vi "EnFlo_TubingCorrection_Sub.vi"(4 "Index":i32, 5 "Analysis Info cluster In":T1={"Colour"=0, "Inst type"=enum."Pitot-static tube", "Inst name"="Manometer voltage", "Symbol"="U", "Code name"="", "Extra Info"="U", "Inst Array"=enum."PWA", "U"=0.0, "u^2"=0.0, "u^3"=0.0, "u^4"=0.0, "Skew_u"=0.0, "Kurt_u"=0.0, "Sd Error in Mean"=0.0, "% u'/U"=0.0, "X"=0.0, "Y"=0.0, "Z"=0.0, "Timescale integral Estimate"=0.0, "Sd Error in Variance"=0.0, "Calib File"=path "", "Calib Constants"=[], "Output Position"=FALSE, "Stats"=enum."None", "Av Sampling Rate"=0.0, "Av No of Samples"=0.0, "Total Meas Time (s)"=0.0, "OrigChName"="", "Max value"=0.0, "Min value"=0.0, "Req Sample Rate Hz"=0.0, "Sync Delay Time (s)"=0.0, "Ch No"=0, "Device"="", "Use Latest Calib"=FALSE, "Port"="", "Metadata Ch Names"=[], "Metadata Ch Values"=[], "Label"="", "chState"=enum."No Selection", "Point Drift"=0.0, "inputConfig"=""} {"Kurt_u" format="%_3g"; "u^4" format="%_3g"; "u^3" format="%_3g"; "Sd Error in Variance" format="%_3g"; "u^2" format="%_3g"; "Sd Error in Mean" format="%_3g"; "U" format="%_3g"; "Sync Delay Time (s)" format="%.4f"; "Total Meas Time (s)" format="%_5g"; "Skew_u" format="%_3g"; "% u'/U" format="%_3g"}, 6 "Time Trace In":T5, 7 "Phase":dbl[](array[numeric]), 8 "Gain":dbl[](array[numeric]), 9 "Freq Hz":dbl[](array[numeric])) -> (0 "Time Trace out":T5, 3 "Analysis Info cluster Out":T1={"Colour"=0, "Inst type"=enum."Pitot-static tube", "Inst name"="Manometer voltage", "Symbol"="U", "Code name"="", "Extra Info"="U", "Inst Array"=enum."PWA", "U"=0.0, "u^2"=0.0, "u^3"=0.0, "u^4"=0.0, "Skew_u"=0.0, "Kurt_u"=0.0, "Sd Error in Mean"=0.0, "% u'/U"=0.0, "X"=0.0, "Y"=0.0, "Z"=0.0, "Timescale integral Estimate"=0.0, "Sd Error in Variance"=0.0, "Calib File"=path "", "Calib Constants"=[], "Output Position"=FALSE, "Stats"=enum."None", "Av Sampling Rate"=0.0, "Av No of Samples"=0.0, "Total Meas Time (s)"=0.0, "OrigChName"="", "Max value"=0.0, "Min value"=0.0, "Req Sample Rate Hz"=0.0, "Sync Delay Time (s)"=0.0, "Ch No"=0, "Device"="", "Use Latest Calib"=FALSE, "Port"="", "Metadata Ch Names"=[], "Metadata Ch Values"=[], "Label"="", "chState"=enum."No Selection", "Point Drift"=0.0, "inputConfig"=""} {"Kurt_u" format="%_3g"; "u^4" format="%_3g"; "u^3" format="%_3g"; "Sd Error in Variance" format="%_3g"; "u^2" format="%_3g"; "Sd Error in Mean" format="%_3g"; "U" format="%_3g"; "Sync Delay Time (s)" format="%.4f"; "Total Meas Time (s)" format="%_5g"; "Skew_u" format="%_3g"; "% u'/U" format="%_3g"})   [LabVIEW 2022 SP3]
uses:
  <vilib>/Analysis/NI_AALPro.lvlib
  <vilib>/Analysis/2dsp.llb/Real FFT.vi
  <vilib>/Analysis/2dsp.llb/Inverse Real FFT.vi
  <vilib>/Analysis/NI_AALBase.lvlib
  <vilib>/Analysis/baseanly.llb/Mean (DBL).vi
  Globals/Meas_global.vi
  Controls/Time_Trace_Cluster.ctl
  Controls/Inst_type.ctl
  Controls/Instrument_Array.ctl
  Controls/Analysis_info_cluster.ctl
  Controls/channelState.ctl
panel:
  out "N Smoothing":i32
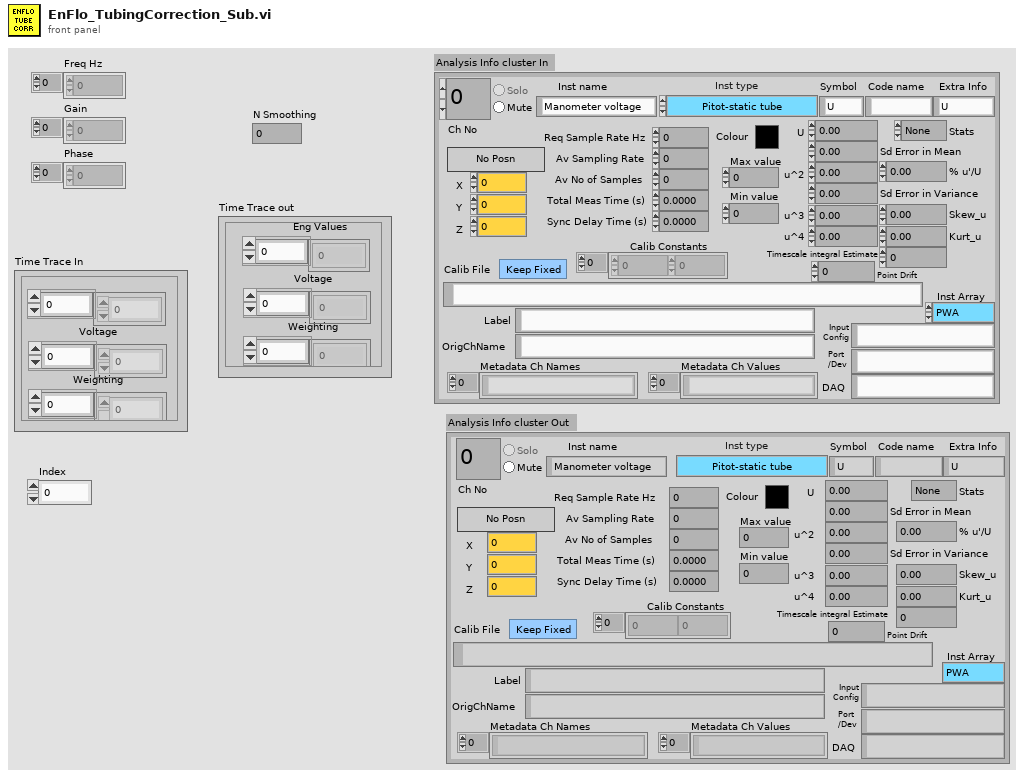
[diagram p1: front panel]
types:
  T1 = typedef "Analysis_info_cluster.ctl" = cluster{"Colour":u32, "Inst type":T2, "Inst name":string, "Symbol":string, "Code name":string, "Extra Info":string, "Inst Array":T3, "U":dbl, "u^2":dbl, "u^3":dbl, "u^4":dbl, "Skew_u":dbl, "Kurt_u":dbl, "Sd Error in Mean":dbl, "% u'/U":dbl, "X":dbl, "Y":dbl, "Z":dbl, "Timescale integral Estimate":dbl, "Sd Error in Variance":dbl, "Calib File":path, "Calib Constants":dbl[], "Output Position":bool, "Stats":enum16{"None", "Basic", "Full"}, "Av Sampling Rate":dbl, "Av No of Samples":dbl, "Total Meas Time (s)":dbl, "OrigChName":string, "Max value":dbl, "Min value":dbl, "Req Sample Rate Hz":dbl, "Sync Delay Time (s)":dbl, "Ch No":i16, "Device":string, "Use Latest Calib":bool, "Port":string, "Metadata Ch Names":string[], "Metadata Ch Values":string[], "Label":string, "chState":T4, "Point Drift":dbl, "inputConfig":string}
  T2 = typedef "Inst_type.ctl" = enum16{"Raw voltage", "Raw with zero offsetting", "Propeller anemometer", "Pressure Transducer", "Pitot-static tube", "Hot wire", "Cross wire 1", "Cross wire 2", "Generic Linear", "Generic Polynomial", "Generic BackPoly", "Fast FID", "Thermocouple", "Cold wire", "Pulsed Wire", "LDA Vel", "LDA Tran time", "LDA Arr time", "Microphone"}
  T3 = typedef "Instrument_Array.ctl" = enum16{"PWA", "LDA", "Analogue"}
  T4 = typedef "channelState.ctl" = enum32{"No Selection", "Solo", "Mute"}
  T5 = typedef "Time_Trace_Cluster.ctl" = cluster{"Weighting":dbl[], "Voltage":dbl[], "Eng Values":dbl[]}
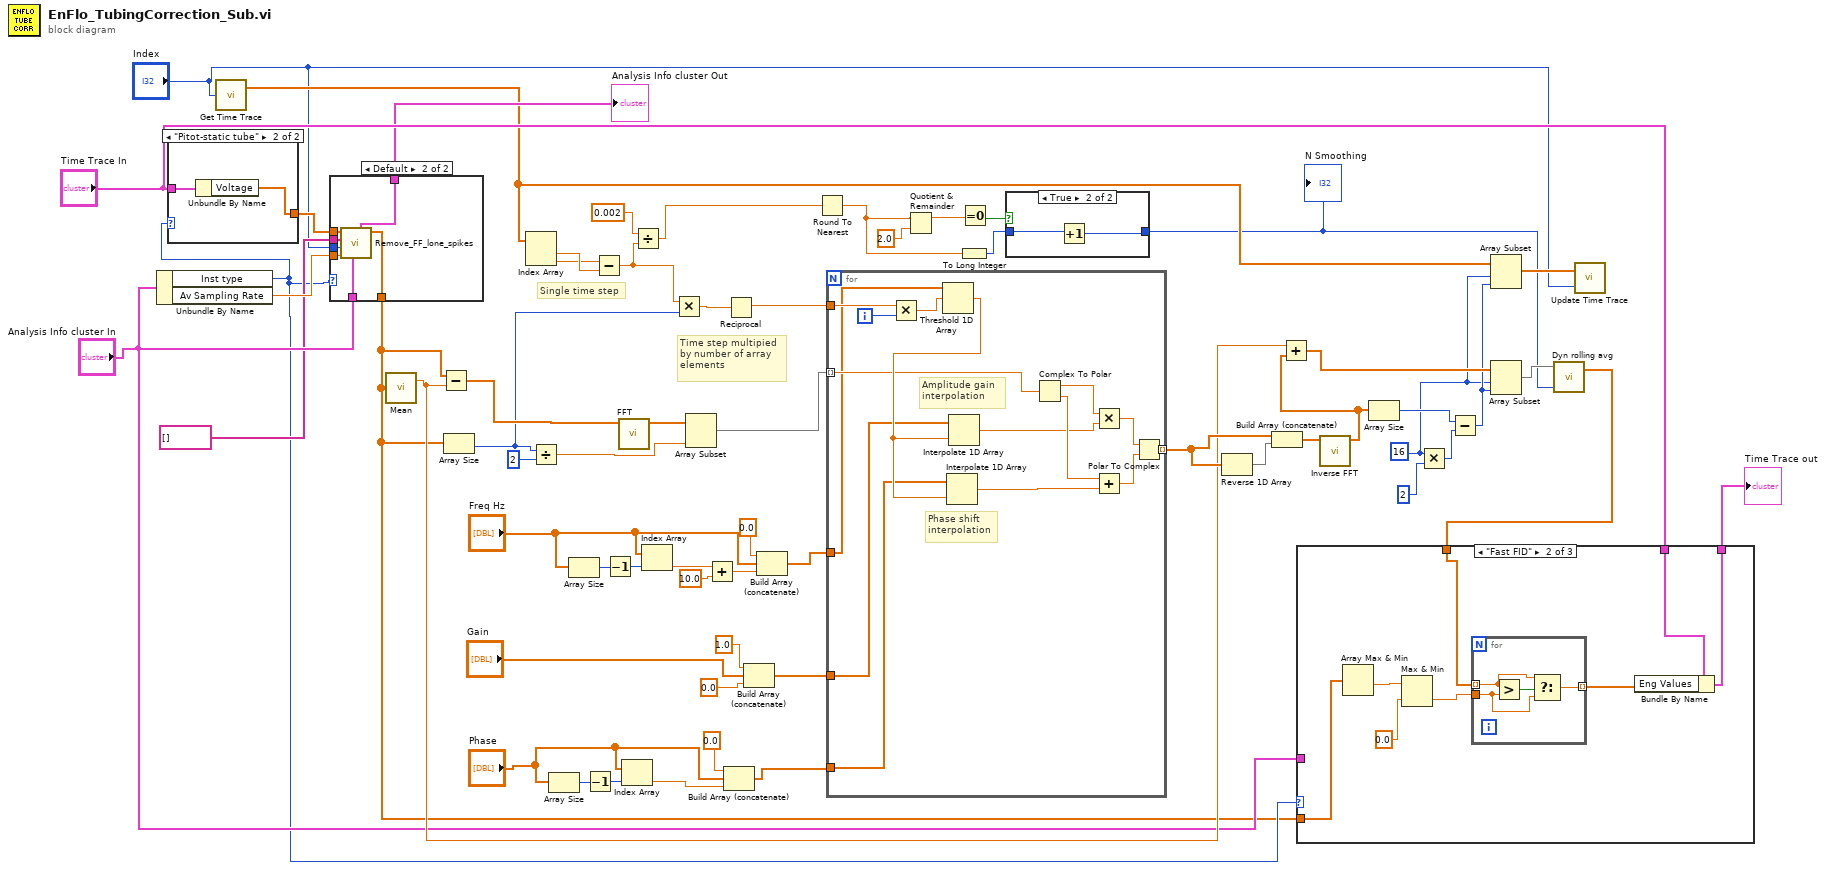
[diagram p0: block diagram]
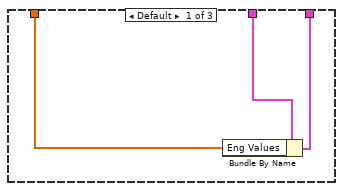
[diagram p4: hidden frame]
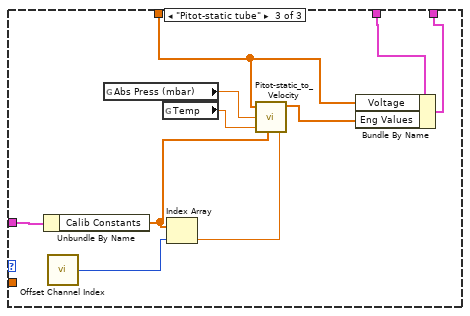
[diagram p5: hidden frame]
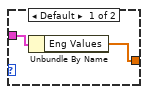
[diagram p6: hidden frame]
diagram:
  w26 = 16
  # "Time step multipied\nby number of array\nelements"
  # "Single time step"
  n1 = Unbundle By Name("Analysis Info cluster In") -> ("Inst type"=w15:T2, "Av Sampling Rate"=w18:dbl)
  n2 = case shown="\"Pitot-static tube\"" w15 {
    tunnel: "Time Trace In" -> [w64 w66]
    tunnel: [w63 w65] -> w25
    frame Default {
      n3 = Unbundle By Name(w64) -> ("Eng Values"=w63:dbl[])
    }
    frame "Pitot-static tube" {
      n4 = Unbundle By Name(w66) -> ("Voltage"=w65:dbl[])
    }
  }
  n5 = call "Get Time Trace.vi"("Channel Index"="Index") -> ("Time (s)"=w20:dbl[])  [unwired: 1 out]
  n6 = case shown="Default" w15 {
    tunnel: w25 -> [w68 w75]
    tunnel: [w68 w74] -> w1
    tunnel: "Analysis Info cluster In" -> [w67 w73]
    tunnel: [w67 w72] -> w21
    tunnel: w18 -> [_ w71]
    tunnel: string[] [] ("Per Block Plug Ins") -> [_ w70]
    tunnel: "Index" -> [_ w69]
    frame "Fast FID" {
    }
    frame Default {
      n7 = call "Remove_FF_lone_spikes.vi"("Analysis Info cluster In"=w73, "Average Sampling Rate"=w71, "index of element"=w69, "Per Block Plug Ins"=w70, "Time Trace"=w75) -> ("Filtered Time Trace"=w74:dbl[], "Analysis Info cluster Out"=w72:T1)  [unwired: 3 in]
    }
  }
  "Analysis Info cluster Out" <- w21
  n8 = call-poly <vilib>:"Mean.vi"("X"=w1) -> ("mean"=w50:dbl)  [unwired: 1 out]
  n9 = Subtract(x=w1, y=w50) -> (x-y=w52:dbl[])
  n10 = Array Size(array=w1) -> (size(s)=w51:i32)
  n11 = Index Array(array=w20) -> (element #1=w60:dbl, element #2=w59:dbl)  [unwired: 2 in]
  n12 = Divide(x=w51, y=2) -> (x/y=w57:dbl)
  n13 = Array Size(array="Phase") -> (size(s)=w43:i32)
  n14 = Array Size(array="Freq Hz") -> (size(s)=w48:i32)
  n15 = Decrement(x=w43) -> (x-1=w42:i32)
  n16 = Subtract(x=w59, y=w60) -> (x-y=w5:dbl)
  n17 = Decrement(x=w48) -> (x-1=w49:i32)
  n18 = call-poly <vilib>:"FFT.vi"("X"=w52) -> ("FFT {X}"=w61:cdb[])  [unwired: 9 in, 1 out]
  n19 = Index Array(array="Phase", index=w42) -> (element=w39:dbl)
  n20 = Divide(x=0.002, y=w5) -> (x/y=w3:dbl)
  n21 = Index Array(array="Freq Hz", index=w49) -> (element=w13:dbl)
  n22 = Multiply(x=w5, y=w51) -> (x*y=w58:dbl)
  n23 = Array Subset(array=w61, length=w57) -> (w56:cdb[])  [unwired: 1 in]
  n24 = Add(x=w13, y=10.0) -> (x+y=w46:dbl)
  n25 = Build Array (concatenate)(0.0, "Phase", w39) -> (w40:dbl[])
  n26 = Reciprocal(x=w58) -> (1/x=w12:dbl)
  n27 = Build Array (concatenate)(1.0, "Gain", 0.0) -> (w38:dbl[])
  n28 = Build Array (concatenate)(0.0, "Freq Hz", w46) -> (w44:dbl[])
  n29 = Round To Nearest(number=w3) -> (nearest integer value=w8:dbl)
  n30 = for {
    tunnel: w12 -> [w90]
    tunnel: w38 -> [w87]
    tunnel: w40 -> [w86]
    tunnel: w56 -> [w85] mode=indexing
    tunnel: [w79] -> w53 mode=indexing
    tunnel: w44 -> [w76]
    i -> [w89]
    # "Phase shift\ninterpolation"
    # "Amplitude gain\ninterpolation"
    n31 = Multiply(x=w90, y=w89) -> (x*y=w77:dbl)
    n32 = Threshold 1D Array(2:w77, 3:w76) -> (0:w88:dbl)  [unwired: 1 in]
    n33 = Interpolate 1D Array(1:w88, 2:w86) -> (0:w82:dbl)
    n34 = Interpolate 1D Array(1:w88, 2:w87) -> (0:w78:dbl)
    n35 = Complex To Polar(r * e^(i*theta)=w85) -> (r=w84:dbl, theta=w83:dbl)
    n36 = Multiply(x=w84, y=w78) -> (x*y=w81:dbl)
    n37 = Add(x=w83, y=w82) -> (x+y=w80:dbl)
    n38 = Polar To Complex(1:w80, 2:w81) -> (0:w79:cdb)
  }
  n39 = Quotient & Remainder(x=w8, y=2.0) -> (x-y*floor(x/y)=w10:dbl)  [unwired: 1 out]
  n40 = To Long Integer(number=w8) -> (32bit integer=w7:i32)
  n41 = Equal To 0?(x=w10) -> (x = 0?=w9:bool)
  n42 = case shown="True" w9 {
    tunnel: [w91 w92] -> w2
    tunnel: w7 -> [w91 w93]
    frame False {
    }
    frame True {
      n43 = Increment(x=w93) -> (x+1=w92:i32)
    }
  }
  "N Smoothing" <- w2
  n44 = Reverse 1D Array(array=w53) -> (reversed array=w55:cdb[])
  n45 = Build Array (concatenate)(w53, w55) -> (w54:cdb[])
  n46 = call-poly <vilib>:"Inverse FFT.vi"("FFT {X}"=w54) -> ("X"=w32:dbl[])  [unwired: 9 in, 1 out]
  n47 = Add(x=w50, y=w32) -> (x+y=w28:dbl[])
  n48 = Array Size(array=w32) -> (size(s)=w29:i32)
  n49 = Multiply(x=w26, y=2) -> (x*y=w30:i32)
  n50 = Subtract(x=w29, y=w30) -> (x-y=w27:i32)
  n51 = Array Subset(array=w20, index=w26, length=w27) -> (w19:dbl[])
  n52 = Array Subset(array=w28, index=w26, length=w27) -> (w14:dbl[])
  n53 = call "Dyn rolling avg.vi"("N"=w2, "orig array"=w14) -> ("moving centered avg"=w6:dbl[])  [unwired: 2 in]
  n54 = case shown="\"Fast FID\"" w15 {
    tunnel: w6 -> [w95 w98 w110]
    tunnel: "Analysis Info cluster In" -> [_ _ w116]
    tunnel: "Time Trace In" -> [w96 w104 w112]
    tunnel: [w94 w103 w111] -> w23
    tunnel: w1 -> [_ w102 _]
    frame Default {
      n55 = Bundle By Name(cluster=w96, "Eng Values"=w95) -> (w94:T5)
    }
    frame "Fast FID" {
      n56 = Array Max & Min(array=w102) -> (min value=w101:dbl)  [unwired: 3 out]
      n57 = Max & Min(x=w101, y=0.0) -> (min(x,y)=w99:dbl)  [unwired: 1 out]
      n58 = for {
        tunnel: w99 -> [w106]
        tunnel: w98 -> [w107] mode=indexing
        tunnel: [w105] -> w97 mode=indexing
        n59 = Greater?(x=w107, y=w106) -> (0:w108:bool)
        n60 = Select(t=w107, s=w108, f=w106) -> (s? t:f=w105:dbl)
      }
      n61 = Bundle By Name(cluster=w104, "Eng Values"=w97) -> (w103:T5)
    }
    frame "Pitot-static tube" {
      n62 = Unbundle By Name(w116) -> ("Calib Constants"=w113:dbl[])
      n63 = call "Offset Channel Index.vi"() -> ("index"=w115:i32)
      n64 = global read "Meas_global.vi" "Abs Press (mbar)"() -> (w117:dbl)
      n65 = global read "Meas_global.vi" "Temp"() -> (w118:dbl)
      n66 = Index Array(array=w113, index=w115) -> (element=w114:dbl)
      n67 = call "Pitot-static_to_Velocity.vi"("Pressure Trans voltage"=w110, "Atmos Press mbar  (1000)"=w117, "Temp  C  (20)"=w118, "Pressure Trans Calib const"=w113, "Mano Zero"=w114) -> ("Velocity (m/s)"=w109:dbl[])  [unwired: 1 in, 2 out]
      n68 = Bundle By Name(cluster=w112, "Voltage"=w110, "Eng Values"=w109) -> (w111:T5)
    }
  }
  "Time Trace out" <- w23
  n69 = call "Update Time Trace.vi"("Channel Index"="Index", "Time (s)"=w19) -> ()  [unwired: 1 in]
